vi "PA warning message.vi"() -> ()   [LabVIEW 2014]
panel:
  out "String":string
  in  "OK":bool
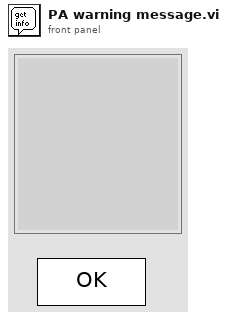
[diagram p1: front panel]
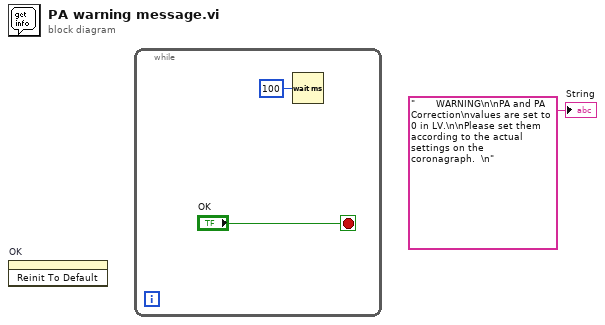
[diagram p0: block diagram]
diagram:
  n1 = invoke on="OK" class="Bool" method="Reinit To Default"() -> ()  [unwired: 3 in, 3 out]
  n2 = while {
    stop <- "OK" stop-if-true
    n3 = Wait (ms)(milliseconds to wait=u32 100) -> ()  [unwired: 1 out]
  }
  "String" <- "       WARNING\n\nPA and PA Correction\nvalues are set to 0 in LV.\n\nPlease set them according to the actual settings on the coronagraph.  \n" ("String")
